vi "greyout_buttons_from_referencearray.vi"(8 "error in (no error)":errorcluster, 10 "Enum":T1=enum."pause", 11 "Array":refnum<vi>[](array[refnum])) -> (0 "error out":errorcluster)   [LabVIEW 2013, in "EMV-Test.lvlib"]
uses:
  EMV-Test.lvlib
  button_states.ctl
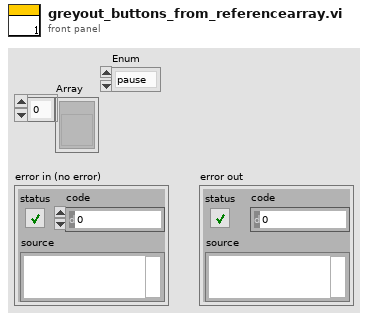
[diagram p1: front panel]
types:
  T1 = typedef "button_states.ctl" = enum16{"ende", "pause", "running", "start"}
  T2 = enum8{"Enabled", "Disabled", "Disabled and Grayed Out"}
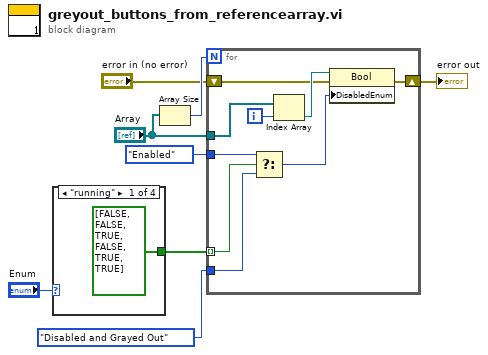
[diagram p0: block diagram]
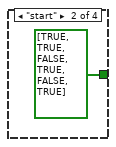
[diagram p2: hidden frame]
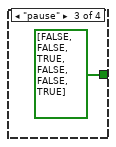
[diagram p3: hidden frame]
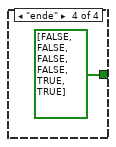
[diagram p4: hidden frame]
diagram:
  n1 = case shown="\"running\"" "Enum" {
    tunnel: [bool[] [FALSE, FALSE, TRUE, FALSE, TRUE, TRUE] bool[] [TRUE, TRUE, FALSE, TRUE, FALSE, TRUE] bool[] [FALSE, FALSE, TRUE, FALSE, FALSE, TRUE] bool[] [FALSE, FALSE, FALSE, FALSE, TRUE, TRUE]] -> w4
    frame "running" {
    }
    frame "start" {
    }
    frame "pause" {
    }
    frame "ende" {
    }
  }
  n2 = Array Size(array="Array") -> (size(s)=w6:i32)
  n3 = for {
    N: w6 -> [_]
    shift-right: [w21] -> w8
    shift-left: "error in (no error)" -> [w17]
    tunnel: "Array" -> [w19]
    tunnel: w4 -> [w15] mode=indexing
    tunnel: T2."Disabled and Grayed Out" ("Disabled") -> [w14]
    tunnel: T2."Enabled" ("f") -> [w13]
    i -> [w20]
    n4 = Select(t=w13, s=w15, f=w14) -> (s? t:f=w16:T2)
    n5 = Index Array(array=w19, index=w20) -> (element=w18:refnum<vi>)
    n6 = property class="Bool"(reference=w18, error in=w17, "DisabledEnum"=w16) -> (error out=w21:errorcluster)  [unwired: 1 out]
  }
  "error out" <- w8
